vi "Test Get Table Names.vi"(11 "Test Case In":refnum<class "Test Open Xml.lvclass">) -> (0 "error out":errorcluster, 3 "Test Case Out":refnum<class "Test Open Xml.lvclass">)   [LabVIEW 2020, in "Test Open Xml.lvclass"]
uses:
  Test Open Xml.lvclass
  Source/Open Xml.lvlib
  0a0d70f3-36fe-46ba-8b3e-e6c07e708d9f.vi
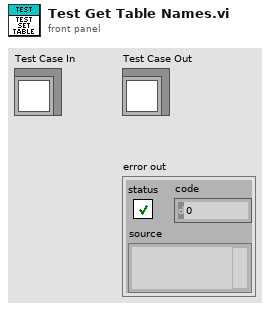
[diagram p1: front panel]
types:
  T1 = cluster{"Sheet Name":string, "Name":string, "Display Name":string, "Range or Cell Address":string}
  T2 = cluster{"Sheet Name":string, "Name":string, "Display Name":string, "Range":string}
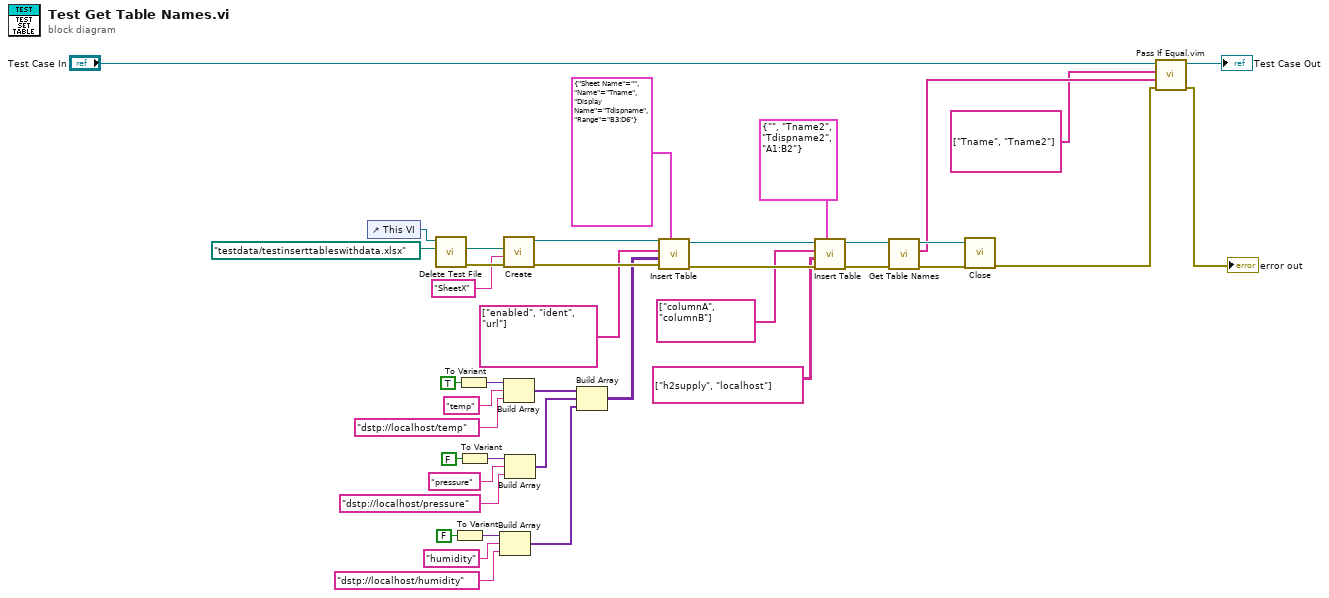
[diagram p0: block diagram]
diagram:
  n1 = control-ref of="This VI"() -> (w31:refnum<vi>)
  n2 = call "Delete Test File.vi"("name or relative path"=path "testdata/testinserttableswithdata.xlsx", "VI in"=w31) -> ("error out"=w32:errorcluster, "deleted path"=w33:path)  [unwired: 8 in]
  n3 = To Variant(anything=FALSE) -> (Variant=w8:variant)
  n4 = To Variant(anything=TRUE) -> (Variant=w17:variant)
  n5 = To Variant(anything=FALSE) -> (Variant=w11:variant)
  n6 = Build Array(w8, "humidity", "dstp://localhost/humidity") -> (w4:variant[])
  n7 = call "Create.vi"("error in"=w32, "SheetName"="SheetX", "Path"=w33) -> ("error out"=w28:errorcluster, "SpreadsheetDoc"=w29:refnum<k24>)  [unwired: 7 in]
  n8 = Build Array(w17, "temp", "dstp://localhost/temp") -> (w14:variant[])
  n9 = Build Array(w11, "pressure", "dstp://localhost/pressure") -> (w5:variant[])
  n10 = Build Array(w14, w5, w4) -> (w3:variant[][])
  n11 = call "Insert Table.vi"("Location"=T2 {"Sheet Name"="", "Name"="Tname", "Display Name"="Tdispname", "Range"="B3:D6"}, "error in"=w28, "Cell Values"=w3, "Header Names"=string[] ["enabled", "ident", "url"], "SpreadsheetDoc in"=w29) -> ("error out"=w35:errorcluster, "SpreadsheetDoc out"=w25:refnum<k24>)  [unwired: 5 in]
  n12 = call "Insert Table.vi"("Location"=T1 {"Sheet Name"="", "Name"="Tname2", "Display Name"="Tdispname2", "Range or Cell Address"="A1:B2"}, "error in"=w35, "Cell Values"=string[][] [["h2supply", "localhost"]], "Header Names"=string[] ["columnA", "columnB"], "SpreadsheetDoc in"=w25) -> ("error out"=w36:errorcluster, "SpreadsheetDoc out"=w1:refnum<k24>)  [unwired: 5 in]
  n13 = call "Get Table Names.vi"("error in"=w36, "SpreadsheetDoc in"=w1) -> ("error out"=w22:errorcluster, "Table Names"=w20:string[], "SpreadsheetDoc out"=w21:refnum<k24>)  [unwired: 6 in, 1 out]
  n14 = call "Close.vi"("error in"=w22, "SpreadsheetDoc"=w21) -> ("error out"=w37:errorcluster)  [unwired: 9 in]
  n15 = call "Pass If Equal.vim"("error in (no error)"=w37, "Actual"=w20, "Expected"=string[] ["Tname", "Tname2"] ("Headers"), "LUnit Test Case In"="Test Case In") -> ("error out"=→"error out":errorcluster, "LUnit Test Case Out"=→"Test Case Out":refnum<class "Test Open Xml.lvclass">)  [unwired: 6 in]
